vi "DAQ_DIO_Open.vi"(0 "reference in":refnum<class "DAQ_Base.lvclass">, 5 "error in (no error)":errorcluster) -> (14 "reference out":refnum<class "DAQ_Base.lvclass">, 19 "error out":errorcluster)   [LabVIEW 2020, in "DAQ_Base.lvclass"]
uses:
  DAQ_Base.lvclass
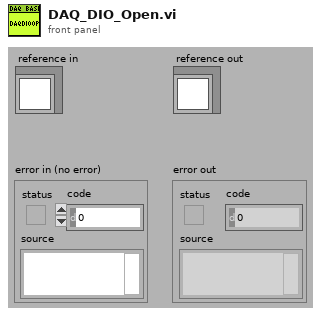
[diagram p1: front panel]
types:
  T1 = typedef "DAQ_Base.lvclass/ObjectAttributesRef.ctl" = refnum<data-value>
  T2 = typedef "DAQ_Base.lvclass/ObjectAttributes.ctl" = cluster{"MyAttribute":dbl, "RootPath":path, "DAQSettings":T3, "DaqCollector":cluster{"CollectDataQueue":refnum<queue>, "ArryDataCollectorChannel":T9[], "RealTimeValues":dbl[]}, "CollectorChannelEnable":bool[]}
  T3 = typedef "DAQ_Base.lvclass/DAQSettings.ctl" = cluster{"SampleSettings":T4, "AI_ChannelSettings":T5, "AO_ChannelSettings":T7, "Cnt_ChannelSettings":T8}
  T4 = typedef "DAQ_Base.lvclass/SampleSettings.ctl" = cluster{"samples per channel":i32, "SampleRate":dbl, "TansMaxLength":dbl, "ReadTimeOut":dbl, "时钟源":tag}
  T5 = typedef "DAQ_Base.lvclass/AI_ChannelSettings.ctl" = cluster{"AI_SettingsArry":cluster{"DeviceName":tag, "physical channels":tag, "AssignName":string, "输入信号类型":T6, "Max_value":dbl, "Min_value":dbl, "单位":i32, "shunt resistor location":i32, "external shunt resistor value":dbl, "标定系数":cluster{"Scale":dbl, "Offset":dbl}}[]}
  T6 = typedef "AI信号类型.ctl" = i32
  T7 = typedef "DAQ_Base.lvclass/AO_ChannelSettings.ctl" = cluster{"布尔":bool}
  T8 = typedef "DAQ_Base.lvclass/Cnt_ChannelSettings.ctl" = cluster{"Cnt_ChannelSettings":cluster{"类型":enum16{"Linear", "Rotate"}, "CounterNbr":tag, "AssignName":string, "单位":u16, "decoding type":u16, "PPR_DistancePerPulse":dbl, "Initial Position ":dbl, "z index enable":bool, "z index phase":i32, "source":tag}[]}
  T9 = typedef "DAQ_Base.lvclass/DataCollector.ctl" = cluster{"DataCollectArry":dbl[][], "Update":bool}
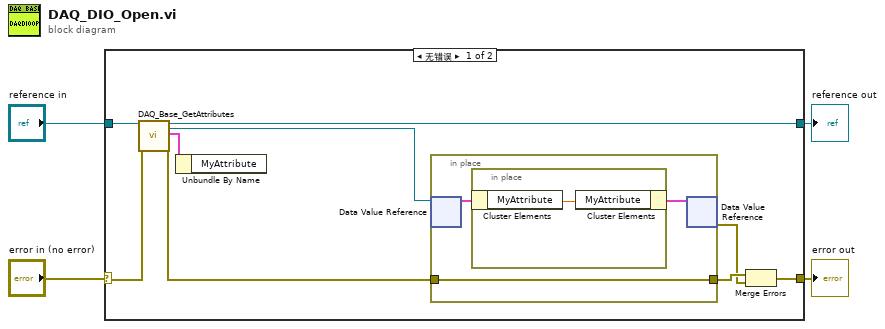
[diagram p0: block diagram]
diagram:
  n1 = case shown="无错误" "error in (no error)" {
    selector: "error in (no error)" -> [w10 w19]
    tunnel: [w13 w19] -> w3
    tunnel: [w11 w18] -> w1
    tunnel: "reference in" -> [w12 w18]
    frame No Error {
      n2 = call "DAQ_Base_GetAttributes.vi"("reference in"=w12, "error in (no error)"=w10) -> ("reference out"=w11:refnum<class "DAQ_Base.lvclass">, "attributes ref"=w5:T1, "attributes"=w8:T2, "error out"=w9:errorcluster)  [unwired: 14 in]
      n3 = Unbundle By Name(w8) -> ()  [unwired: 1 out]
      n4 = in-place {
        in-place-border: w9 -> [w14]
        in-place-border: [w14] -> w7
        n5 = in-place-dvr #1(w5) -> (w15:T2)  [unwired: 1 out]
        n6 = in-place {
          n7 = in-place-cluster #2(w15) -> ("MyAttribute"=w17:dbl)
          n8 = in-place-cluster #2("MyAttribute"=w17) -> (w16:T2)
        }
        n9 = in-place-dvr #1(w16) -> (w6:errorcluster)  [unwired: 1 out]
      }
      n10 = Merge Errors(w7, w6) -> (w13:errorcluster)
    }
    frame Error {
    }
  }
  "error out" <- w3
  "reference out" <- w1
